vi "UnscentedKalmanFilter_Transform.vi"(3 "ResidualFuncExtra":variant, 4 "Dim":i32, 5 "residualFunc":T2, 6 "S":i32, 7 "MeanFuncExtra":variant, 8 "Wc":T1, 9 "Wm":T1, 10 "Sigmas":T1, 11 "MeanFunc":T2) -> (0 "Error":bool, 1 "P":T1, 2 "X":T1)   [LabVIEW 2019, in "Trajectory_Library.lvlib"]
doc: "Creates a new LINEAR SYSTEM data cluster with the specified values. \n\n\nInputs: \n - XXX -- XXX.\n\nOutputs:\n - XXX -- XXX."
uses:
  Trajectory_Library.lvlib
  CALLBACK_FUNC_TYPE.ctl
  <vilib>/Analysis/Matrix/Datatypes/RealMatrix.ctl
  <vilib>/Analysis/baseanly.llb/Real A x B.vi
  <vilib>/Analysis/7linalg.llb/Real Transpose Matrix.vi
  MatrixHelper_CoerceSize.vi
  <vilib>/Analysis/NI_AALBase.lvlib
  <vilib>/Analysis/NI_AALPro.lvlib
  <vilib>/Analysis/Matrix/NI_Matrix.lvlib
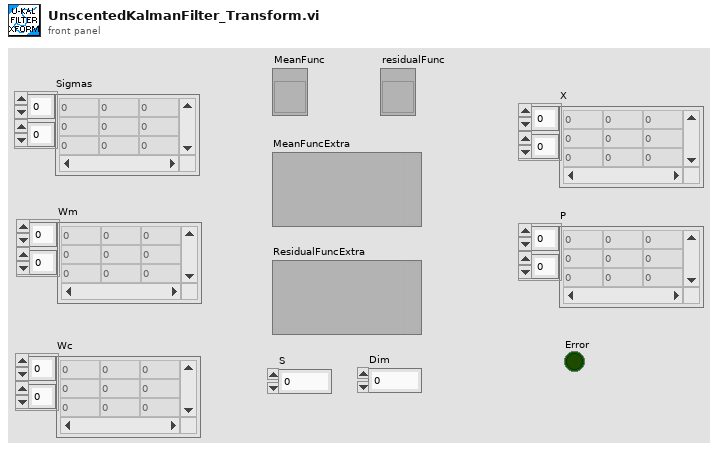
[diagram p1: front panel]
types:
  T1 = typedef "NI_Matrix.lvlib/RealMatrix.ctl" = dbl[][]
  T2 = typedef "Trajectory_Library.lvlib/CALLBACK_FUNC_TYPE.ctl" = refnum<vi>
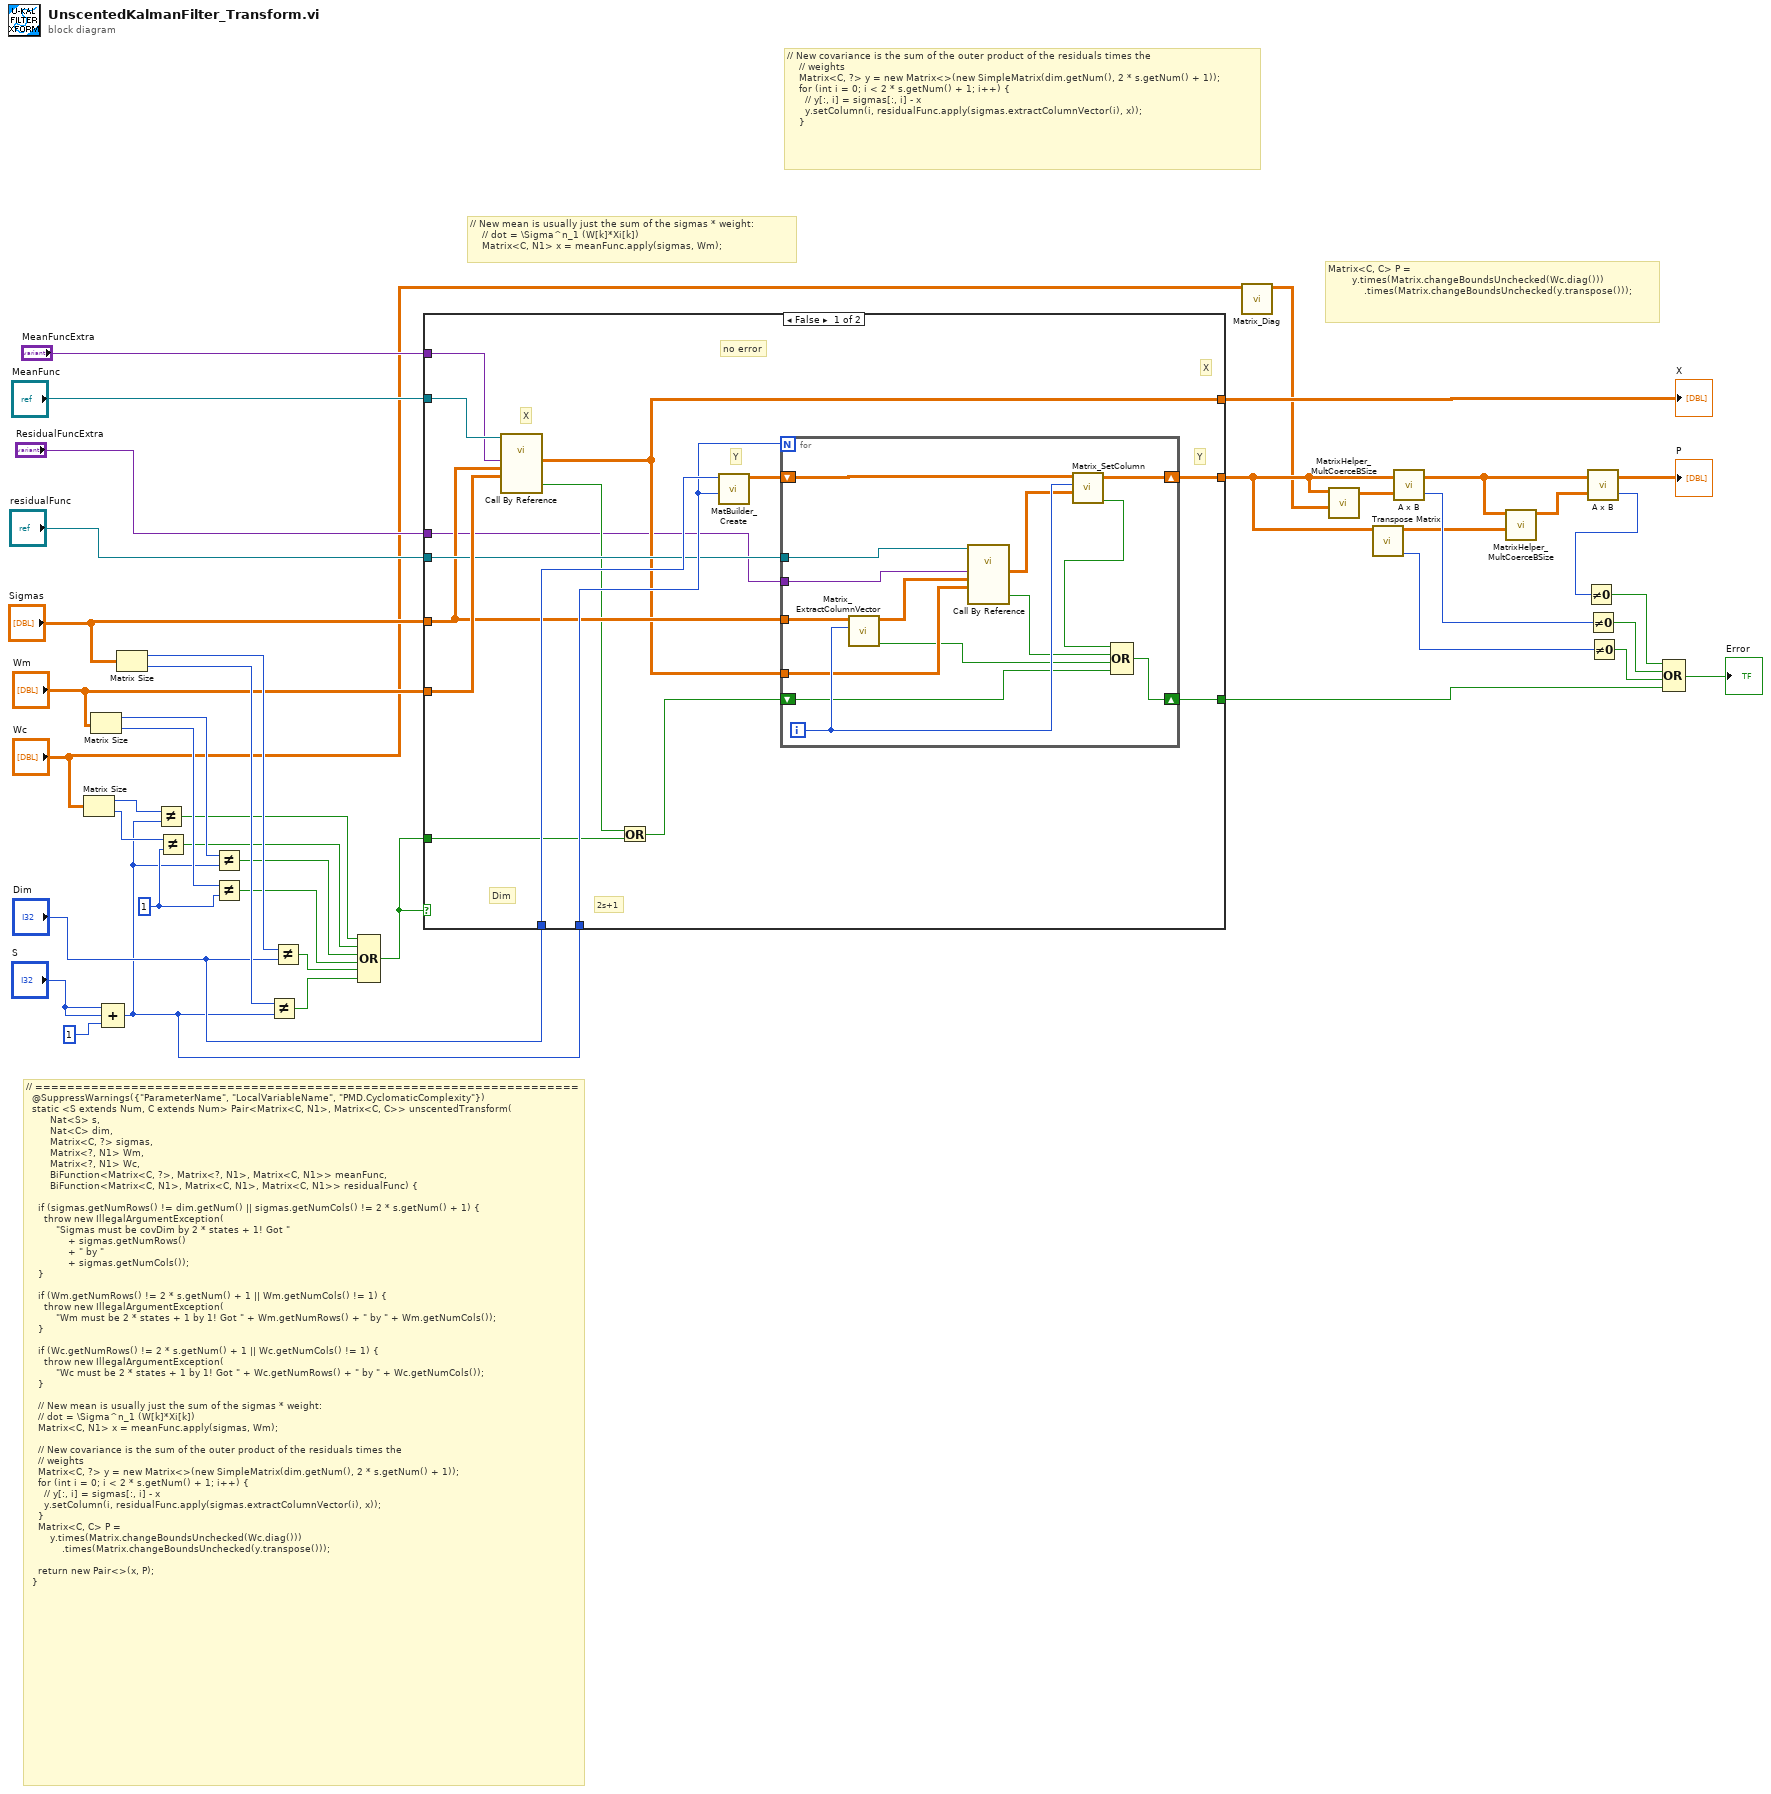
[diagram p0: block diagram]
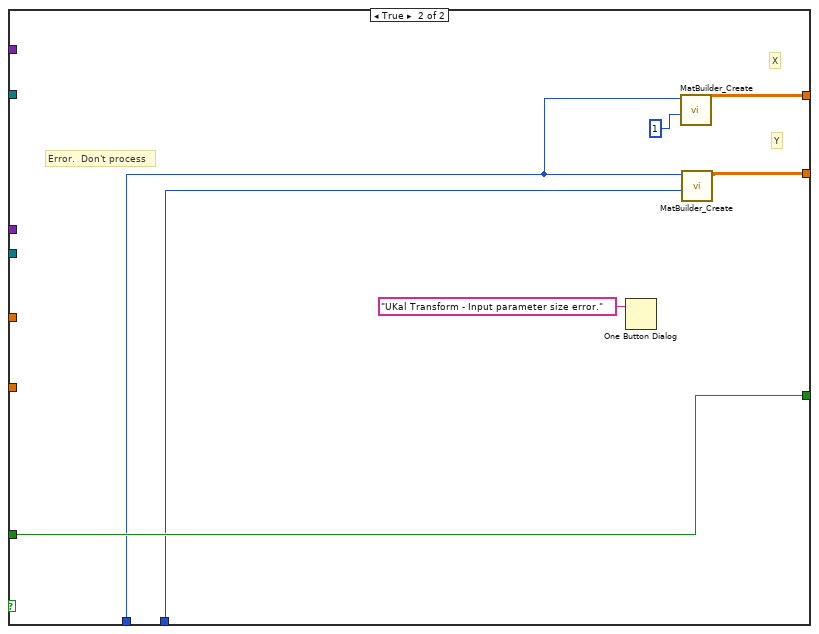
[diagram p2: hidden frame]
diagram:
  w30 = 1 ("y")
  # "Matrix<C, C> P =\n        y.times(Matrix.changeBoundsUnchecked(Wc.diag()))\n            .times(Matrix.changeBoundsUnchecked(y.transpose()));"
  # "// New mean is usually just the sum of the sigmas * weight:\n    // dot = \\Sigma^n_1 (W[k]*Xi[k])\n    Matrix<C, N1> x = meanFunc.apply(sigmas, Wm);"
  # "// New covariance is the sum of the outer product of the residuals times the\n    // weights\n    Matrix<C, ?> y = new Matrix<>(new SimpleMatrix(dim.getNum(), 2 * s.getNum() + 1));\n    for (int i = 0; i < 2 * s.getNum() + 1; i++) {\n      // y[:, i] = sigmas[:, i] - x\n      y.setColumn(i, residualFunc.apply(sigmas.extractColumnVector(i), x));\n    }"
  # "// ====================================================================\n  @SuppressWarnings({\"ParameterName\", \"LocalVariableName\", \"PMD.CyclomaticComplexity\"})\n  static <S extends Num, C extends Num> Pair<Matrix<C, N1>, Matrix<C, C>> unscentedTransform(\n      \t\tNat<S> s,\n      \t\tNat<C> dim,\n      \t\tMatrix<C, ?> sigmas,\n      \t\tMatrix<?, N1> Wm,\n      \t\tMatrix<?, N1> Wc,\n      \t\tBiFunction<Matrix<C, ?>, Matrix<?, N1>, Matrix<C, N1>> meanFunc,\n      \t\tBiFunction<Matrix<C, N1>, Matrix<C, N1>, Matrix<C, N1>> residualFunc) {\n\n    if (sigmas.getNumRows() != dim.getNum() || sigmas.getNumCols() != 2 * s.getNum() + 1) {\n      throw new IllegalArgumentException(\n          \"Sigmas must be covDim by 2 * states + 1! Got \"\n              + sigmas.getNumRows()\n              + \" by \"\n              + sigmas.getNumCols());\n    }\n\n    if (Wm.getNumRows() != 2 * s.getNum() + 1 || Wm.getNumCols() != 1) {\n      throw new IllegalArgumentException(\n          \"Wm must be 2 * states + 1 by 1! Got \" + Wm.getNumRows() + \" by \" + Wm.getNumCols());\n    }\n\n    if (Wc.getNumRows() != 2 * s.getNum() + 1 || Wc.getNumCols() != 1) {\n      throw new IllegalArgumentException(\n          \"Wc must be 2 * states + 1 by 1! Got \" + Wc.getNumRows() + \" by \" + Wc.getNumCols());\n    }\n\n    // New mean is usually just the sum of the sigmas * weight:\n    // dot = \\Sigma^n_1 (W[k]*Xi[k])\n    Matrix<C, N1> x = meanFunc.apply(sigmas, Wm);\n\n    // New covariance is the sum of the outer product of the residuals times the\n    // weights\n    Matrix<C, ?> y = new Matrix<>(new SimpleMatrix(dim.getNum(), 2 * s.getNum() + 1));\n    for (int i = 0; i < 2 * s.getNum() + 1; i++) {\n      // y[:, i] = sigmas[:, i] - x\n      y.setColumn(i, residualFunc.apply(sigmas.extractColumnVector(i), x));\n    }\n    Matrix<C, C> P =\n        y.times(Matrix.changeBoundsUnchecked(Wc.diag()))\n            .times(Matrix.changeBoundsUnchecked(y.transpose()));\n\n    return new Pair<>(x, P);\n  }"
  n1 = Matrix Size(0:"Wc") -> (1:w31:i32, 2:w29:i32)
  n2 = Matrix Size(0:"Wm") -> (1:w35:i32, 2:w34:i32)
  n3 = Compound Arithmetic op=ADD("S", "S", 1 ("value")) -> (w22:i32)
  n4 = Matrix Size(0:"Sigmas") -> (1:w41:i32, 2:w38:i32)
  n5 = Not Equal?(x=w31, y=w22) -> (x != y?=w27:bool)
  n6 = Not Equal?(x=w29, y=w30) -> (x != y?=w28:bool)
  n7 = Not Equal?(x=w35, y=w22) -> (x != y?=w32:bool)
  n8 = Not Equal?(x=w34, y=w30) -> (x != y?=w33:bool)
  n9 = Not Equal?(x=w38, y=w22) -> (x != y?=w37:bool)
  n10 = Not Equal?(x=w41, y="Dim") -> (x != y?=w36:bool)
  n11 = Compound Arithmetic op=OR(w27, w28, w32, w33, w36, w37) -> (w20:bool)
  n12 = case shown="False" w20 {
    tunnel: "Sigmas" -> [w50 _]
    tunnel: "Wm" -> [w55 _]
    tunnel: "MeanFunc" -> [w56 _]
    tunnel: "Dim" -> [w54 w73]
    tunnel: w22 -> [w53 w76]
    tunnel: "residualFunc" -> [w51 _]
    tunnel: w20 -> [w48 w77]
    tunnel: [w46 w74] -> w19
    tunnel: [w45 w77] -> w12
    tunnel: [w44 w75] -> w4
    tunnel: "MeanFuncExtra" -> [w43 _]
    tunnel: "ResidualFuncExtra" -> [w42 _]
    frame False {
      # "Y"
      # "no error"
      # "Y"
      # "X"
      # "X"
      # "2s+1"
      # "Dim"
      n13 = call-by-ref "?"(reference=w56, "U"=w55, "X"=w50, "Variant"=w43) -> ("Error"=w49:bool, "NewX"=w46:T1)  [unwired: 8 in, 2 out]
      n14 = Or(x=w49, y=w48) -> (x .or. y?=w47:bool)
      n15 = call "MatBuilder_Create.vi"("Columns"=w53, "Rows"=w54) -> ("output matrix"=w52:T1)  [unwired: 9 in]
      n16 = for {
        N: w53 -> [_]
        shift-right: [w62] -> w44
        shift-left: w52 -> [w70]
        tunnel: w51 -> [w69]
        tunnel: w50 -> [w68]
        tunnel: w46 -> [w65]
        shift-right: [w61] -> w45
        shift-left: w47 -> [w64]
        tunnel: w42 -> [w60]
        i -> [w67]
        n17 = call "Matrix_ExtractColumnVector.vi"("Column"=w67, "input matrix"=w68) -> ("Error"=w58:bool, "output column"=w66:T1)  [unwired: 8 in]
        n18 = call-by-ref "?"(reference=w69, "U"=w65, "X"=w66, "Variant"=w60) -> ("Error"=w59:bool, "NewX"=w63:T1)  [unwired: 8 in, 2 out]
        n19 = call "Matrix_SetColumn.vi"("Fill Vector"=w63, "Column"=w67, "input matrix"=w70) -> ("Error"=w57:bool, "output matrix"=w62:T1)  [unwired: 7 in]
        n20 = Compound Arithmetic op=OR(w57, w59, w58, w64) -> (w61:bool)
      }
    }
    frame True {
      # "Y"
      # "X"
      # "Error.  Don't process"
      n21 = One Button Dialog(message="UKal Transform - Input parameter size error.") -> ()  [unwired: 1 in, 1 out]
      n22 = call "MatBuilder_Create.vi"("Columns"=1, "Rows"=w73) -> ("output matrix"=w74:T1)  [unwired: 9 in]
      n23 = call "MatBuilder_Create.vi"("Columns"=w76, "Rows"=w73) -> ("output matrix"=w75:T1)  [unwired: 9 in]
    }
  }
  "X" <- w19
  n24 = call "Matrix_Diag.vi"("input matrix"="Wc") -> ("output matrix"=w1:T1)  [unwired: 10 in]
  n25 = call "MatrixHelper_MultCoerceBSize.vi"("B"=w1, "A"=w4) -> ("Updated B"=w3:T1)  [unwired: 8 in, 1 out]
  n26 = call-poly <vilib>:"Transpose Matrix.vi"("Input Matrix"=w4) -> ("error"=w16:i32, "Matrix Transpose"=w6:T1)  [unwired: 9 in]
  n27 = call-poly <vilib>:"A x B.vi"("B"=w3, "A"=w4) -> ("error"=w17:i32, "A x B"=w7:T1)
  n28 = call "MatrixHelper_MultCoerceBSize.vi"("B"=w6, "A"=w7) -> ("Updated B"=w5:T1)  [unwired: 8 in, 1 out]
  n29 = call-poly <vilib>:"A x B.vi"("B"=w5, "A"=w7) -> ("error"=w18:i32, "A x B"=→"P":T1)
  n30 = Not Equal To 0?(x=w18) -> (x != 0?=w15:bool)
  n31 = Not Equal To 0?(x=w17) -> (x != 0?=w14:bool)
  n32 = Not Equal To 0?(x=w16) -> (x != 0?=w13:bool)
  n33 = Compound Arithmetic op=OR(w15, w14, w13, w12) -> (→"Error":bool)
